vi "test-DiffDrvPoseEst2-next-gaussian-rand.vi"(8 "Init":bool, 11 "Multiplier":dbl=1.0) -> (3 "Gaussian white noise":dbl)   [LabVIEW 2019]
uses:
  <vilib>/ptbypt/NI_PtbyPt.lvlib
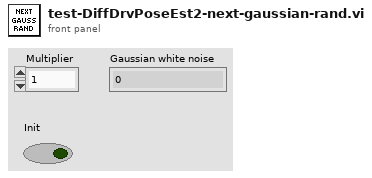
[diagram p1: front panel]
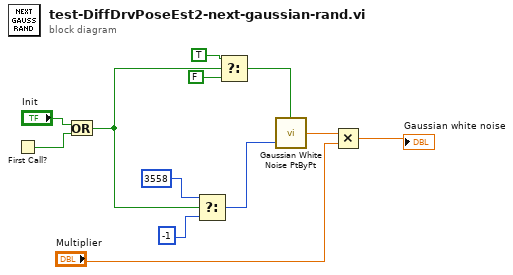
[diagram p0: block diagram]
diagram:
  n1 = First Call?() -> (First Call?: T/F=w2:bool)
  n2 = Or(x="Init", y=w2) -> (x .or. y?=w1:bool)
  n3 = Select(t=3558 ("seed"), s=w1, f=-1 ("seed")) -> (s? t:f=w7:i32)
  n4 = Select(t=TRUE, s=w1, f=FALSE) -> (s? t:f=w10:bool)
  n5 = call <vilib>:"Gaussian White Noise PtByPt.vi"("initialize"=w10, "seed"=w7) -> ("Gaussian white noise"=w6:dbl)  [unwired: 1 in]
  n6 = Multiply(x=w6, y="Multiplier") -> (x*y=→"Gaussian white noise":dbl)
